vi "get_data.vi"(0 "data buffer":i8[](array[numeric])) -> (1 "Click Value":i8, 2 "X Value":i8, 3 "Y Value":i8)   [LabVIEW 2012]
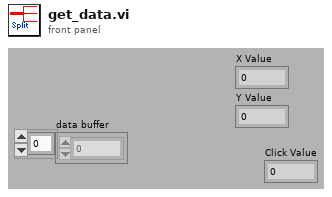
[diagram p1: front panel]
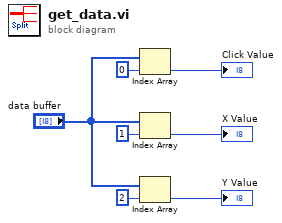
[diagram p0: block diagram]
diagram:
  n1 = Index Array(array="data buffer", index=0) -> (element=→"Click Value":i8)
  n2 = Index Array(array="data buffer", index=1) -> (element=→"X Value":i8)
  n3 = Index Array(array="data buffer", index=2) -> (element=→"Y Value":i8)
